vi "Configure Sequencer Trigger Source Catalog.vi"(8 "error in (no error)":errorcluster, 10 "Instance (1)":i32=1, 11 "VISA resource name":refnum<visa-resource-name>) -> (0 "error out":errorcluster, 2 "Catalog":string, 3 "VISA resource name out":refnum<visa-resource-name>)   [LabVIEW 2020, in "Rohde&Schwarz CMXP GPRF.lvlib"]
doc: "Queries all available trigger source strings.\n\nAttribute:\nRSCMXPGPRF_ATTR_SEQUENCER_TRIGGER_SOURCE_CATALOG\n\nRemote-control command:\nTRIGger:GPRF:GEN<i>:SEQuencer:ISTRigger:CATalog?"
uses:
  <instrlib>/Rohde&Schwarz CMXP GPRF/Rohde&Schwarz CMXP GPRF.lvlib
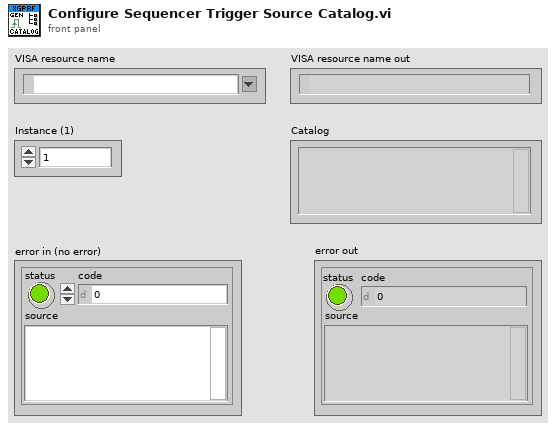
[diagram p1: front panel]
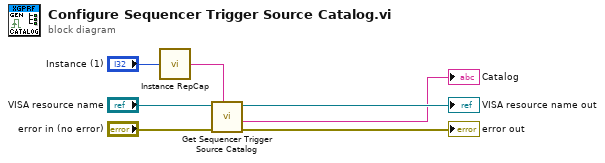
[diagram p0: block diagram]
diagram:
  n1 = call <instrlib>:"Instance RepCap.vi"("Instance in"="Instance (1)") -> ("Instance out"=w7:string)
  n2 = call "Get Sequencer Trigger Source Catalog"("Repeated Capabilities"=w7, "error in (no error)"="error in (no error)", "instrument handle"="VISA resource name") -> ("error out"=→"error out":errorcluster, "Sequencer Trigger Source Catalog"=→"Catalog":string, "instrument handle out"=→"VISA resource name out":refnum<visa-resource-name>)  [unwired: 6 in]
